vi "TriggerHandling.vi"() -> ()   [LabVIEW 2014]
uses:
  <vilib>/eio/EIONode/EIONode.xnode
  <vilib>/platform/TimedLoop/XDataNode/XDataNode.xnode
  <vilib>/Platform/TimedLoop/XDataNode/nitl_modes.ctl
  <vilib>/Platform/TimedLoop/XDataNode/XDNodeRunTimeDep.lvlib
  <vilib>/Platform/TimedLoop/XDataNode/wakeup.ctl
  <vilib>/Platform/TimedLoop/XDataNode/timing_clust.ctl
  <vilib>/rvi/eio/common/nirviEmuTemplateMethod_errors.vi
panel:
  out "C3DIGIN":bool
  out "C2DIGIN":bool
  out "C0DIGIN":bool
  out "C1DIGIN":bool
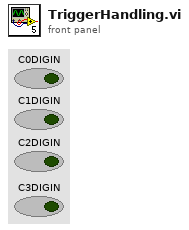
[diagram p1: front panel]
types:
  T1 = typedef "XDNodeRunTimeDep.lvlib/timing_clust.ctl" = cluster{"Expected End [f-1]":u64, "Actual End [f-1]":u64, "Finished Late? [f-1]":bool, "Expected End [i-1]":u64, "Actual End [i-1]":u64, "Finished Late? [i-1]":bool, "Expected Start [i]":u64, "Actual Start [i]":u64, "Expected Start [f]":u64, "Actual Start [f]":u64, "Source Name":string, "Structure Name":string, "Period":i64, "Deadline":i64, "Offset":i64, "Start":i64, "Priority":i32, "Timeout":i32, "Mode":T2, "Wakeup Reason":T3, "Error":errorcluster, "Source Type":string, "Secondary Source Type":string, "Global End Time":u64, "Global Start Time":u64, "Frame Duration":u64, "Iteration Duration":u64, "Assigned CPU":i32, "I/O Scan Engine Mode":u32}
  T2 = typedef "XDNodeRunTimeDep.lvlib/nitl_modes.ctl" = enum32{"No Change", "Process missed periods, maintain original phase", "Discard missed periods, maintain original phase", "Process missed periods, ignore original phase", "Discard missed periods, ignore original phase"}
  T3 = typedef "XDNodeRunTimeDep.lvlib/wakeup.ctl" = enum32{"Normal", "Aborted", "Asynchronous wakeup", "Timing source error", "Timed loop error", "Timeout"}
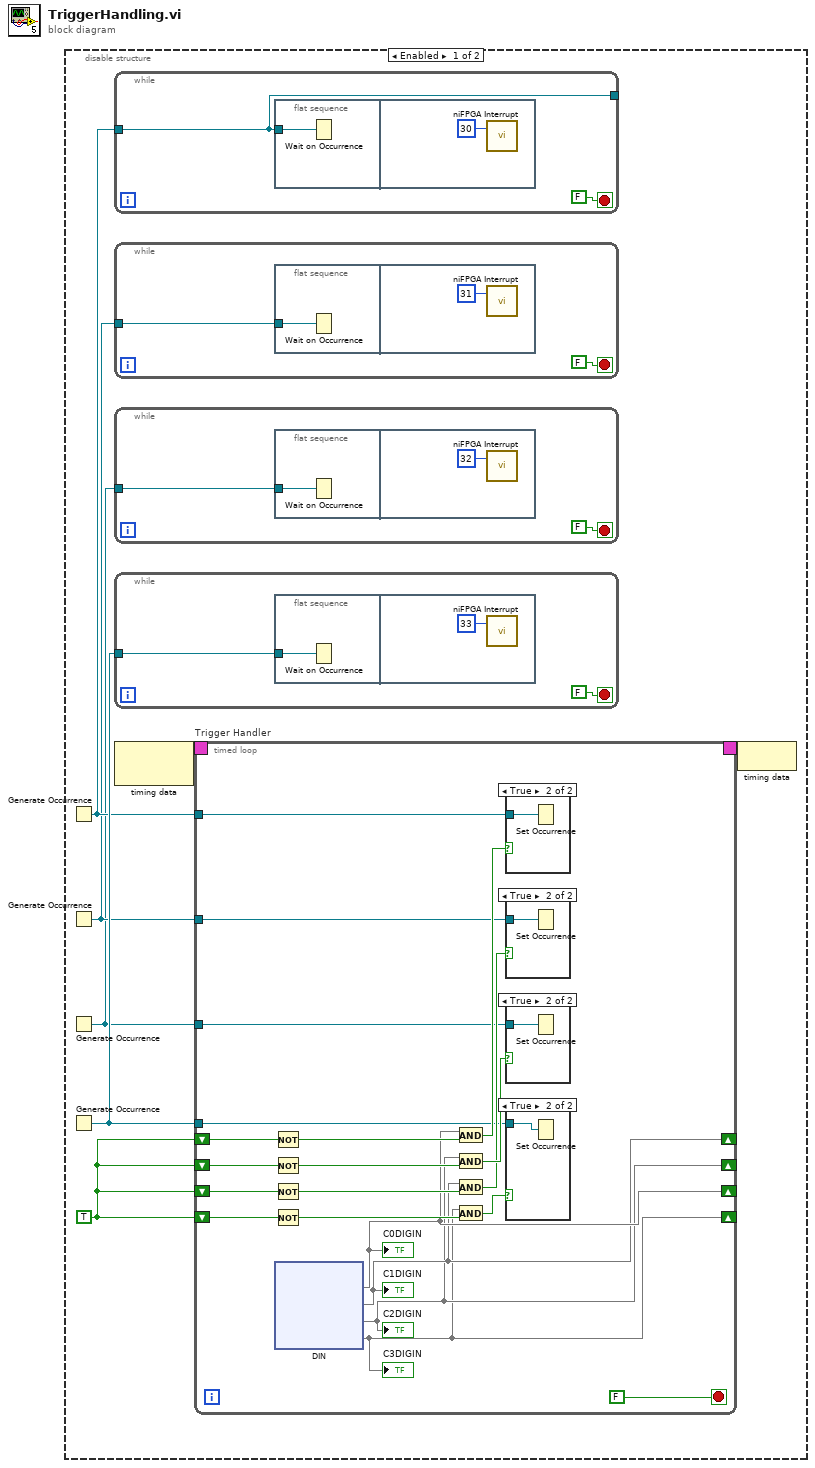
[diagram p0: block diagram]
diagram:
  n1 = disable-structure shown="Enabled" {
    frame Enabled {
      w1 = TRUE
      n2 = Generate Occurrence() -> (w4:refnum<k4>)
      n3 = Generate Occurrence() -> (w3:refnum<k4>)
      n4 = Generate Occurrence() -> (w2:refnum<k4>)
      n5 = Generate Occurrence() -> (w5:refnum<k4>)
      n6 = while {
        tunnel: [w8] -> _
        tunnel: w4 -> [w8]
        stop <- FALSE stop-if-true
        n7 = flat-sequence {
          tunnel: w8 -> [w10]
          frame #0 {
            n8 = Wait on Occurrence(2:w10) -> ()  [unwired: 2 in, 1 out]
          }
          frame #1 {
            n9 = call <vilib>:"niFPGA Interrupt.vi"("IRQ Number (0)"=u8 30 ("IRQ Bit (0-31)")) -> ()  [unwired: 2 in]
          }
        }
      }
      n10 = while {
        tunnel: w3 -> [w12]
        stop <- FALSE stop-if-true
        n11 = flat-sequence {
          tunnel: w12 -> [w14]
          frame #0 {
            n12 = Wait on Occurrence(2:w14) -> ()  [unwired: 2 in, 1 out]
          }
          frame #1 {
            n13 = call <vilib>:"niFPGA Interrupt.vi"("IRQ Number (0)"=u8 31 ("IRQ Bit (0-31)")) -> ()  [unwired: 2 in]
          }
        }
      }
      n14 = while {
        tunnel: w2 -> [w16]
        stop <- FALSE stop-if-true
        n15 = flat-sequence {
          tunnel: w16 -> [w18]
          frame #0 {
            n16 = Wait on Occurrence(2:w18) -> ()  [unwired: 2 in, 1 out]
          }
          frame #1 {
            n17 = call <vilib>:"niFPGA Interrupt.vi"("IRQ Number (0)"=u8 32 ("IRQ Bit (0-31)")) -> ()  [unwired: 2 in]
          }
        }
      }
      n18 = while {
        tunnel: w5 -> [w20]
        stop <- FALSE stop-if-true
        n19 = flat-sequence {
          tunnel: w20 -> [w22]
          frame #0 {
            n20 = Wait on Occurrence(2:w22) -> ()  [unwired: 2 in, 1 out]
          }
          frame #1 {
            n21 = call <vilib>:"niFPGA Interrupt.vi"("IRQ Number (0)"=u8 33 ("IRQ Bit (0-31)")) -> ()  [unwired: 2 in]
          }
        }
      }
      n22 = node-c288() -> (w7:T1)  [unwired: 1 in]
      n23 = timed-loop "Trigger Handler" {
        shift-right: [w24] -> _
        shift-left: w1 -> [w42]
        shift-right: [w25] -> _
        shift-left: w1 -> [w40]
        shift-right: [w26] -> _
        shift-left: w1 -> [w36]
        shift-right: [w27] -> _
        shift-left: w1 -> [w37]
        tunnel: w4 -> [w31]
        timing: w7 -> [_]
        timing-out: [_] -> w6
        tunnel: w3 -> [w30]
        tunnel: w2 -> [w29]
        tunnel: w5 -> [w28]
        stop <- FALSE stop-if-true
        n24 = Not(x=w36) -> (.not. x?=w38:bool)
        n25 = Not(x=w40) -> (.not. x?=w41:bool)
        n26 = Not(x=w37) -> (.not. x?=w39:bool)
        n27 = Not(x=w42) -> (.not. x?=w43:bool)
        n28 = xnode "DIN"() -> ("C0DIGIN"=w27, "C1DIGIN"=w26, "C2DIGIN"=w25, "C3DIGIN"=w24)  [unwired: 4 in, 4 out]
        "C1DIGIN" <- w26
        "C0DIGIN" <- w27
        "C2DIGIN" <- w25
        "C3DIGIN" <- w24
        n29 = And(x=w27, y=w38) -> (x .and. y?=w32:bool)
        n30 = And(x=w25, y=w41) -> (x .and. y?=w34:bool)
        n31 = And(x=w26, y=w39) -> (x .and. y?=w33:bool)
        n32 = And(x=w24, y=w43) -> (x .and. y?=w35:bool)
        n33 = case shown="True" w32 {
          tunnel: w31 -> [_ w45]
          frame False {
          }
          frame True {
            n34 = Set Occurrence(w45) -> ()
          }
        }
        n35 = case shown="True" w33 {
          tunnel: w30 -> [_ w48]
          frame False {
          }
          frame True {
            n36 = Set Occurrence(w48) -> ()
          }
        }
        n37 = case shown="True" w34 {
          tunnel: w29 -> [_ w46]
          frame False {
          }
          frame True {
            n38 = Set Occurrence(w46) -> ()
          }
        }
        n39 = case shown="True" w35 {
          tunnel: w28 -> [_ w47]
          frame False {
          }
          frame True {
            n40 = Set Occurrence(w47) -> ()
          }
        }
      }
      n41 = node-c288(w6) -> ()
    }
    frame Disabled {
    }
  }
